vi "PISetPosition.vi"(0 "Current Position (µm)":cluster{"x":dbl, "y":dbl, "z":dbl} {"z" format="%.2f"; "y" format="%.2f"; "x" format="%.2f"}) -> ()   [LabVIEW 2009]
uses:
  <vilib>/Daq/1easyio.llb/AO Update Channels (scaled array).vi
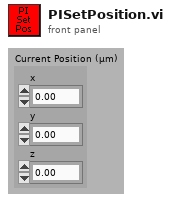
[diagram p1: front panel]
types:
  T1 = typedef "AnalogSettings.ctt" = cluster{"PCI 671x Device Number":u32, "Samples per Unit":u32}
  T2 = typedef "StageSettings.ctt" = cluster{"channels (x, y, z)":tag, "Stage Scaling (V/µm)":dbl}
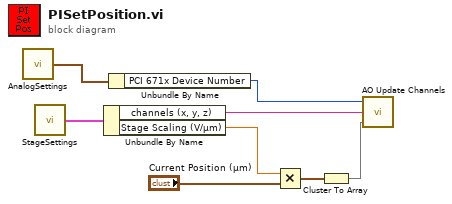
[diagram p0: block diagram]
diagram:
  n1 = call "AnalogSettings.vi"() -> ("Analog Settings (output)"=w6:T1)  [unwired: 2 in]
  n2 = call "StageSettings.vi"() -> ("PI Stage Setup (output)"=w8:T2)  [unwired: 2 in]
  n3 = Unbundle By Name(w8) -> ("channels (x, y, z)"=w2:tag, "Stage Scaling (V/µm)"=w5:dbl)
  n4 = Unbundle By Name(w6) -> ("PCI 671x Device Number"=w3:u32)
  n5 = Multiply(x=w5, y="Current Position (µm)") -> (x*y=w4:cluster{"x":dbl, "y":dbl, "z":dbl})
  n6 = Cluster To Array(cluster=w4) -> (array=w7:dbl[])
  n7 = call-poly <vilib>:"AO Update Channels.vi"("values"=w7, "channels (0)"=w2, "device"=w3) -> ()
